vi "RT Message handler loop.vi"(9 "Message handler data":T3, 11 "RT Queues":T5) -> (1 "stop button":bool)   [LabVIEW 2018]
uses:
  Type Defs/Queues cluster.ctl
  ICL-LabVIEW_General/Message Scheduler/message scheduler.lvclass
  Type Defs/Message loop data.ctl
  Type Defs/FPGA reference.ctl
  Type Defs/RT Status.ctl
  ICL-LabVIEW_General/Message Scheduler/generic message queue/standard message queue/standard message.lvclass
  C:/GitHub/ICL-LabVIEW_General/Message Scheduler/generic message queue/generic message.lvclass
  Queue VIs/De-queue RT message element.vi
  Communications loop/create incident - command.vi
  Queue VIs/En-queue RT data element.vi
  Queue VIs/En-queue RT comms element.vi
  Communications loop/create incident - message.vi
  <vilib>/Utility/error.llb/Error Cluster From Error Code.vi
  Queue VIs/En-queue RT message element.vi
  Queue VIs/En-queue RT FIFO element.vi
  Queue VIs/Close Message queue.vi
  <vilib>/nisyscfg/Close (System).vi
  <vilib>/FPGAPlugInAG/cRIO-9056/niLvFpga_Close_cRIO-9056.vi
  <vilib>/ErrorRing/Error Ring.xnode
  <vilib>/rvi/interface/nirviCloseFPGA/nirviCloseFPGA.xnode
  FPGA Bitfiles/CompressorRigV2_CompressorFPGA_FPGAMainV3_7sPRekuravM.lvbitx
  ICL-LabVIEW_General/Message Scheduler/scheduled message/scheduled message.lvclass
  <vilib>/nisyscfg/nisyscfg.lvlib
  Message Handler loop/FPGA commands/RT - FPGA commands.lvlib
panel:
  out "Interlocks":T1
  out "RT Status":T2
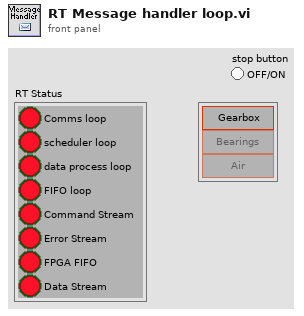
[diagram p1: front panel]
types:
  T1 = cluster{"gearboxOil":bool, "bearingOil":bool, "gearboxAir":bool}
  T2 = typedef "RT Status.ctl" = cluster{"Comms loop":bool, "scheduler loop":bool, "data process loop":bool, "FIFO loop":bool, "Command Stream":bool, "Error Stream":bool, "FPGA FIFO":bool, "Data Stream":bool}
  T3 = typedef "Message loop data.ctl" = cluster{"Parameters":cluster{"FPGA Ref":T4, "configID":u32, "activeChannels":cluster{"index":u16, "name":string}[]}, "Variables":cluster{"RT Status":T2, "watchdog":timestamp, "limitsEnabled":bool, "Interlocks":cluster{"gearboxOil":bool, "bearingOil":bool, "gearboxAir":bool}}}
  T4 = typedef "FPGA reference.ctl" = refnum<k20>
  T5 = typedef "Queues cluster.ctl" = cluster{"RT Message":refnum<queue>, "RT Comms":refnum<queue>, "RT Data":refnum<queue>, "RT FIFO":refnum<queue>, "message scheduler":refnum<class "message scheduler.lvclass">}
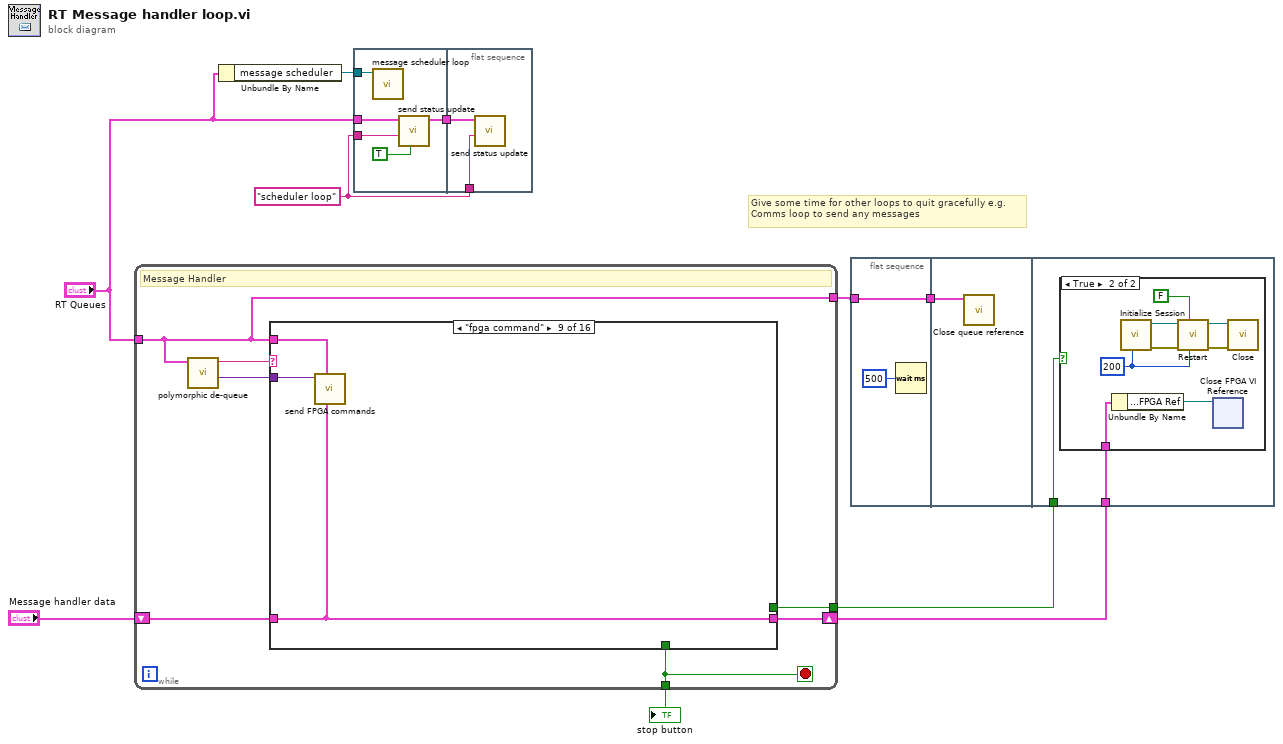
[diagram p0: block diagram]
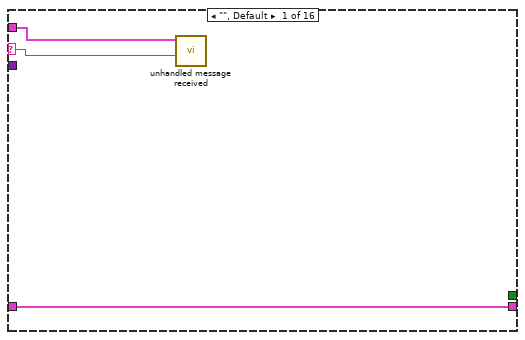
[diagram p3: hidden frame]
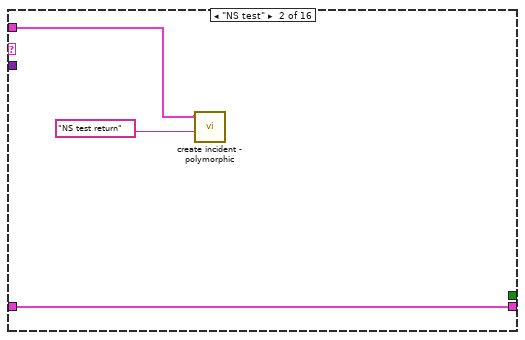
[diagram p4: hidden frame]
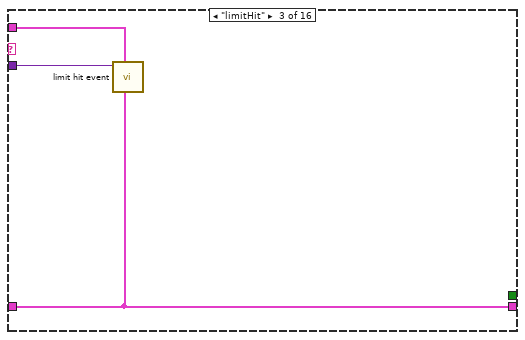
[diagram p5: hidden frame]
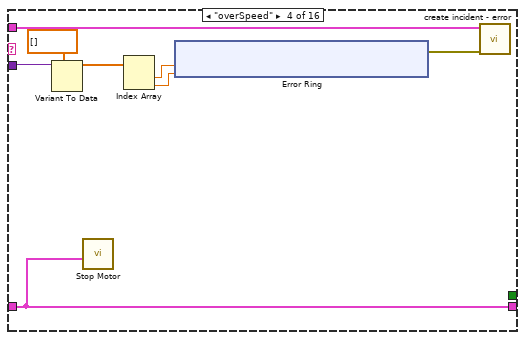
[diagram p6: hidden frame]
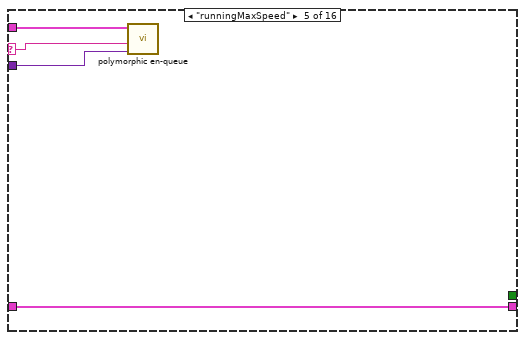
[diagram p7: hidden frame]
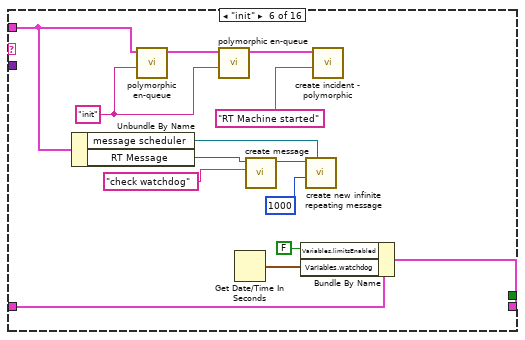
[diagram p8: hidden frame]
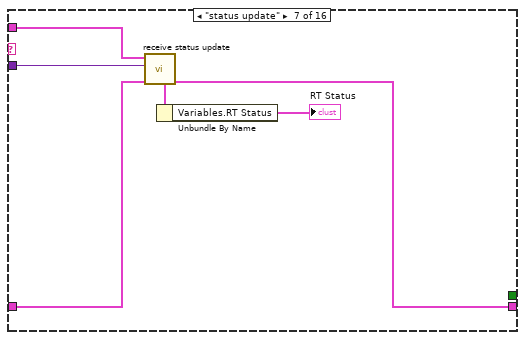
[diagram p9: hidden frame]
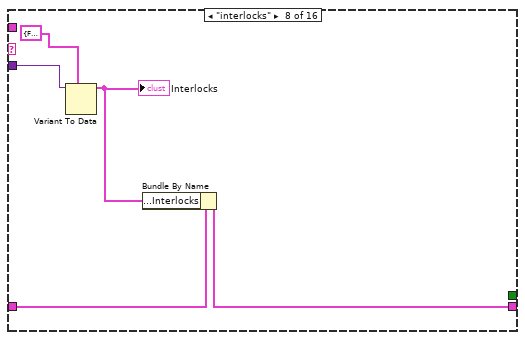
[diagram p10: hidden frame]
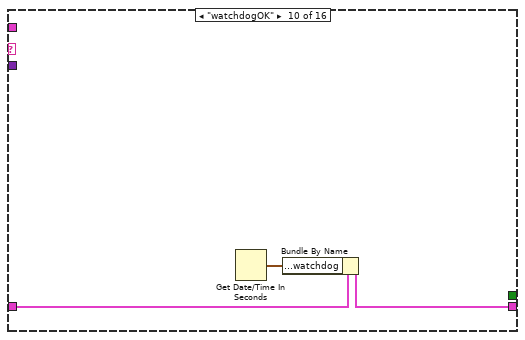
[diagram p11: hidden frame]
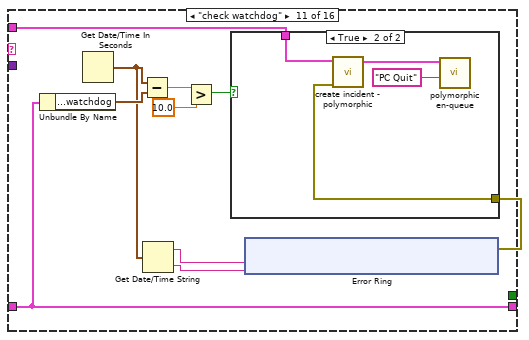
[diagram p12: hidden frame]
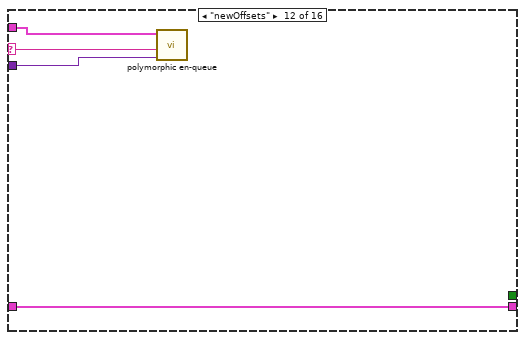
[diagram p14: hidden frame]
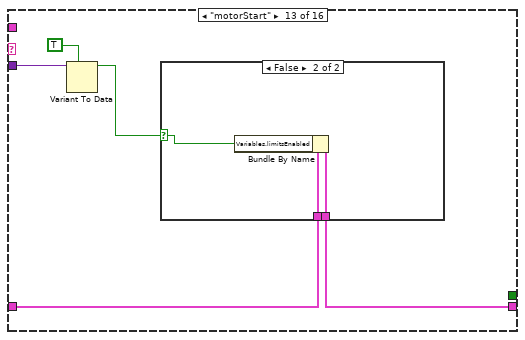
[diagram p15: hidden frame]
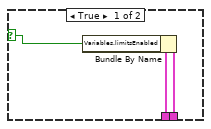
[diagram p16: hidden frame]
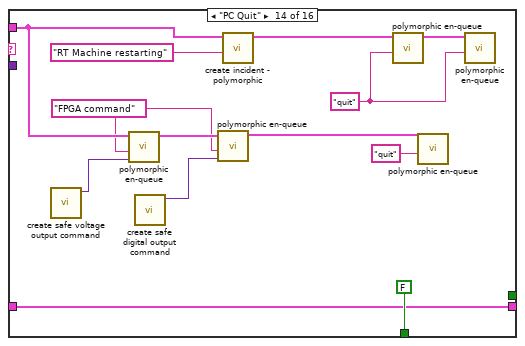
[diagram p17: hidden frame]
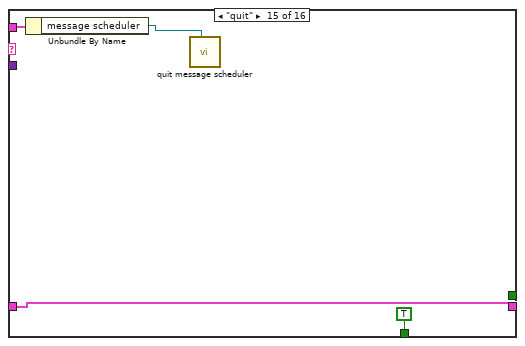
[diagram p18: hidden frame]
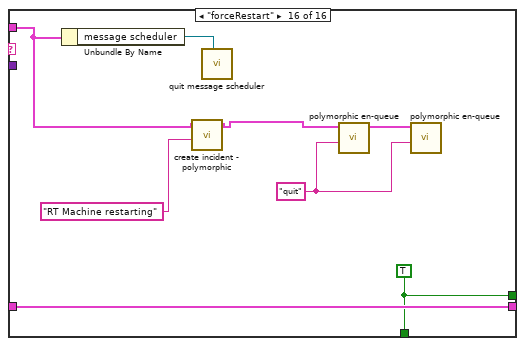
[diagram p19: hidden frame]
diagram:
  w5 = "scheduler loop" ("Message")
  # "Give some time for other loops to quit gracefully e.g. Comms loop to send any messages"
  n1 = while {
    tunnel: "RT Queues" -> [w13]
    shift-right: [w15] -> w8
    shift-left: "Message handler data" -> [w16]
    tunnel: [w13] -> w9
    tunnel: [w12] -> w2
    tunnel: [w11] -> w1
    stop <- w11 stop-if-true
    # "Message Handler"
    n2 = call-poly "polymorphic de-queue.vi"("RT Queues"=w13) -> ("Data"=w14:variant, "Message"=w17:string)  [unwired: 9 in]
    n3 = case shown="\"fpga command\"" w17 {
      selector: w17 -> [w19 _ _ _ w42 _ _ _ _ _ _ w98 _ _ _ _]
      tunnel: w13 -> [w18 w22 w24 w33 w43 w56 w61 _ w69 _ w80 w99 _ w117 w126 w131]
      tunnel: w16 -> [w20 w23 w25 w34 w44 w54 w63 w66 w70 w74 w84 w100 w105 w121 w127 w133]
      tunnel: [w20 w23 w25 w34 w44 w53 w60 w65 w70 w73 w84 w100 w102 w121 w127 w133] -> w15
      tunnel: [_ _ _ _ _ _ _ _ _ _ _ _ _ FALSE TRUE w132] -> w11
      tunnel: w14 -> [_ _ w26 w31 w41 _ w62 w68 w71 _ _ w97 w104 _ _ _]
      tunnel: [_ _ _ _ _ _ _ _ _ _ _ _ _ _ _ w132] -> w12
      frame "", Default {
        n4 = call "unhandled message received.vi"("unhandled message"=w19, "RT Queues"=w18) -> ()  [unwired: 10 in]
      }
      frame "NS test" {
        n5 = call-poly "create incident - polymorphic.vi"("command"="NS test return" ("message"), "RT Queues"=w22) -> ()  [unwired: 10 in]
      }
      frame "limitHit" {
        n6 = call "limit hit event.vi"("Message handler data"=w25, "RT Queues"=w24, "Data"=w26) -> ()  [unwired: 9 in]
      }
      frame "overSpeed" {
        n7 = Variant To Data(type=dbl[] [] ("parameter 0"), Variant=w31) -> (data=w29:dbl[])  [unwired: 1 in, 1 out]
        n8 = call "Stop Motor.vi"("Message handler data"=w34) -> ()  [unwired: 11 in]
        n9 = Index Array(array=w29) -> (element #1=w28:dbl, element #2=w27:dbl)  [unwired: 2 in]
        n10 = xnode "Error Ring"("parameter 0"=w28, "parameter 1"=w27) -> ("error out"=w32:errorcluster)
        n11 = call "create incident - error.vi"("error"=w32, "RT Queues"=w33) -> ()  [unwired: 9 in, 1 out]
      }
      frame "runningMaxSpeed" {
        n12 = call-poly "polymorphic en-queue.vi"("Data"=w41, "Message"=w42, "RT Queues"=w43) -> ()  [unwired: 6 in, 3 out]
      }
      frame "init" {
        w58 = "init" ("Message")
        # "Initialise Variables to safe values (Parameters are passed in already)"
        n13 = Unbundle By Name(w56) -> ("message scheduler"=w55:refnum<class "message scheduler.lvclass">, "RT Message"=w50:refnum<queue>)
        n14 = call-poly "polymorphic en-queue.vi"("Message"=w58, "RT Queues"=w56) -> ("RT Queues out"=w57:T5)  [unwired: 9 in]
        n15 = call-poly "polymorphic en-queue.vi"("Message"=w58, "RT Queues"=w57) -> ("RT Queues out"=w47:T5)  [unwired: 7 in, 2 out]
        n16 = Get Date/Time In Seconds() -> (seconds since 1Jan1904=w52:timestamp)
        n17 = call "create message.vi"("message"="check watchdog", "queue ref"=w50) -> ("standard message out"=w51:refnum<class "standard message.lvclass">)  [unwired: 8 in, 1 out]
        n18 = Bundle By Name(cluster=w54, "Variables.limitsEnabled"=FALSE, "Variables.watchdog"=w52) -> (w53:T3)
        n19 = call "create new infinite repeating message.vi"("message scheduler"=w55, "ms delay"=u32 1000, "message"=w51) -> ()  [unwired: 7 in, 2 out]
        n20 = call-poly "create incident - polymorphic.vi"("message"="RT Machine started" ("Description"), "RT Queues"=w47) -> ()  [unwired: 9 in, 1 out]
      }
      frame "status update" {
        n21 = call "receive status update.vi"("Message handler data in"=w63, "Data"=w62, "RT Queues"=w61) -> ("Message handler data out"=w60:T3)  [unwired: 8 in]
        n22 = Unbundle By Name(w60) -> ("Variables.RT Status"=→"RT Status":T2)
      }
      frame "interlocks" {
        n23 = Variant To Data(type=T1 {"gearboxOil"=FALSE, "bearingOil"=FALSE, "gearboxAir"=FALSE} ("Interlocks"), Variant=w68) -> (data=w64:T1)  [unwired: 1 in, 1 out]
        "Interlocks" <- w64
        n24 = Bundle By Name(cluster=w66, "Variables.Interlocks"=w64) -> (w65:T3)
      }
      frame "fpga command" {
        n25 = call "send FPGA commands.vi"("Message handler data"=w70, "RT Queues"=w69, "Data"=w71) -> ()  [unwired: 9 in]
      }
      frame "watchdogOK" {
        n26 = Get Date/Time In Seconds() -> (seconds since 1Jan1904=w72:timestamp)
        n27 = Bundle By Name(cluster=w74, "Variables.watchdog"=w72) -> (w73:T3)
      }
      frame "check watchdog" {
        n28 = Unbundle By Name(w84) -> ("Variables.watchdog"=w83:timestamp)
        n29 = Get Date/Time In Seconds() -> (seconds since 1Jan1904=w78:timestamp)
        n30 = Subtract(x=w78, y=w83) -> (x-y=w82:dbl)
        n31 = Get Date/Time String(seconds (now)=w78) -> (date string=w77:string, time string=w76:string)  [unwired: 2 in]
        n32 = Greater?(x=w82, y=10.0) -> (0:w79:bool)
        n33 = xnode "Error Ring"("parameter 0"=w77, "parameter 1"=w76) -> ("error out"=w75:errorcluster)
        n34 = case shown="True" w79 {
          tunnel: w80 -> [_ w95]
          tunnel: w75 -> [_ w94]
          frame False {
          }
          frame True {
            n35 = call-poly "create incident - polymorphic.vi"("error"=w94, "RT Queues"=w95) -> ("RT Queues out"=w93:T5)  [unwired: 9 in]
            n36 = call-poly "polymorphic en-queue.vi"("Message"="PC Quit", "RT Queues"=w93) -> ()  [unwired: 9 in, 1 out]
          }
        }
      }
      frame "newOffsets" {
        n37 = call-poly "polymorphic en-queue.vi"("Data"=w97, "Message"=w98, "RT Queues"=w99) -> ()  [unwired: 6 in, 3 out]
      }
      frame "motorStart" {
        n38 = Variant To Data(type=TRUE, Variant=w104) -> (data=w101:bool)  [unwired: 1 in, 1 out]
        n39 = case shown="False" w101 {
          selector: w101 -> [w106 w109]
          tunnel: w105 -> [w108 w111]
          tunnel: [w107 w110] -> w102
          frame True {
            n40 = Bundle By Name(cluster=w108, "Variables.limitsEnabled"=w106) -> (w107:T3)
          }
          frame False {
            n41 = Bundle By Name(cluster=w111, "Variables.limitsEnabled"=w109) -> (w110:T3)
          }
        }
      }
      frame "PC Quit" {
        w112 = "FPGA command" ("Message")
        w122 = "quit" ("Message")
        # "Send quit commands to other loops, destroy open references"
        n42 = call "create safe voltage output command.vi"() -> ("command message"=w116:variant)  [unwired: 11 in]
        n43 = call-poly "polymorphic en-queue.vi"("Data"=w116, "Message"=w112, "RT Queues"=w117) -> ("RT Queues out"=w115:T5)  [unwired: 8 in]
        n44 = call "create safe digital output command.vi"() -> ("command message"=w113:variant)  [unwired: 11 in]
        n45 = call-poly "polymorphic en-queue.vi"("Data"=w113, "Message"=w112, "RT Queues"=w115) -> ("RT Queues out"=w114:T5)  [unwired: 8 in]
        n46 = call-poly "create incident - polymorphic.vi"("message"="RT Machine restarting" ("Description"), "RT Queues"=w117) -> ("RT Queues out"=w118:T5)  [unwired: 9 in]
        n47 = call-poly "polymorphic en-queue.vi"("Message"=w122, "RT Queues"=w118) -> ("RT Queues out"=w123:T5)  [unwired: 9 in]
        n48 = call-poly "polymorphic en-queue.vi"("Message"="quit", "RT Queues"=w114) -> ()  [unwired: 9 in, 1 out]
        n49 = call-poly "polymorphic en-queue.vi"("Message"=w122, "RT Queues"=w123) -> ()  [unwired: 7 in, 3 out]
      }
      frame "quit" {
        n50 = Unbundle By Name(w126) -> ("message scheduler"=w125:refnum<class "message scheduler.lvclass">)
        n51 = call "quit message scheduler.vi"("message scheduler"=w125) -> ()  [unwired: 10 in, 1 out]
      }
      frame "forceRestart" {
        w134 = "quit" ("Message")
        w132 = TRUE
        # "Send quit commands to other loops, destroy open references"
        n52 = Unbundle By Name(w131) -> ("message scheduler"=w136:refnum<class "message scheduler.lvclass">)
        n53 = call-poly "create incident - polymorphic.vi"("message"="RT Machine restarting" ("Description"), "RT Queues"=w131) -> ("RT Queues out"=w130:T5)  [unwired: 9 in]
        n54 = call "quit message scheduler.vi"("message scheduler"=w136) -> ()  [unwired: 10 in, 1 out]
        n55 = call-poly "polymorphic en-queue.vi"("Message"=w134, "RT Queues"=w130) -> ("RT Queues out"=w135:T5)  [unwired: 9 in]
        n56 = call-poly "polymorphic en-queue.vi"("Message"=w134, "RT Queues"=w135) -> ()  [unwired: 7 in, 3 out]
      }
    }
  }
  "stop button" <- w1
  n57 = Unbundle By Name("RT Queues") -> ("message scheduler"=w6:refnum<class "message scheduler.lvclass">)
  n58 = flat-sequence {
    tunnel: w6 -> [w141]
    tunnel: w5 -> [w139]
    tunnel: "RT Queues" -> [w140]
    tunnel: [w137] -> w7
    tunnel: w7 -> [w143]
    tunnel: w5 -> [w142]
    frame #0 {
      n59 = call "message scheduler loop.vi"("message scheduler"=w141) -> ()  [unwired: 11 in]
      n60 = call "send status update.vi"("status (F)"=TRUE, "subject"=w139, "RT Queues"=w140) -> ("RT Queues out"=w137:T5)  [unwired: 8 in]
    }
    frame #1 {
      n61 = call "send status update.vi"("subject"=w142, "RT Queues"=w143) -> ()  [unwired: 9 in, 1 out]
    }
  }
  n62 = flat-sequence {
    tunnel: w9 -> [w145]
    tunnel: [w145] -> w3
    tunnel: w3 -> [w146]
    tunnel: w8 -> [w148]
    tunnel: w2 -> [w147]
    frame #0 {
      n63 = Wait (ms)(milliseconds to wait=u32 500) -> ()  [unwired: 1 out]
    }
    frame #1 {
      n64 = call-poly "Close queue reference.vi"("RT Queues"=w146) -> ()  [unwired: 11 in]
    }
    frame #2 {
      n65 = case shown="True" w147 {
        tunnel: w148 -> [_ w156]
        frame False {
        }
        frame True {
          w150 = u32 200 ("Connect Timeout (4000 ms)")
          n66 = Unbundle By Name(w156) -> ("Parameters.FPGA Ref"=w149:T4)
          n67 = call <vilib>:"Initialize Session.vi"("Connect Timeout (4000 ms)"=w150) -> ("error out"=w154:errorcluster, "Session out"=w155:refnum<k21>)  [unwired: 9 in]
          n68 = call <vilib>:"Restart.vi"("Timeout (180,000 ms)"=w150, "Wait Until Complete (T)"=FALSE, "error in (no error)"=w154, "Session in"=w155) -> ("error out"=w151:errorcluster, "Session out"=w152:refnum<k21>)  [unwired: 5 in, 1 out]
          n69 = xnode "Close FPGA VI Reference"("FPGA VI Reference In"=w149) -> ()  [unwired: 1 in, 1 out]
          n70 = call-poly <vilib>:"Close.vi"("error in (no error)"=w151, "Session in"=w152) -> ()  [unwired: 9 in, 1 out]
        }
      }
    }
  }
